vi "RT_Thrust_Force_in_DLR_Body_Reference_System_2 (SubVI).vi"(6 "Act_b(i)":dbl[](array[numeric]), 8 "Vehicle Parameters":T1, 9 "i":i32, 10 "cluster":T2, 11 "Data":dbl[][](array[numeric])) -> (3 "FE_b":dbl[](array[numeric]))   [LabVIEW 2017]
panel:
  out "Fez":dbl
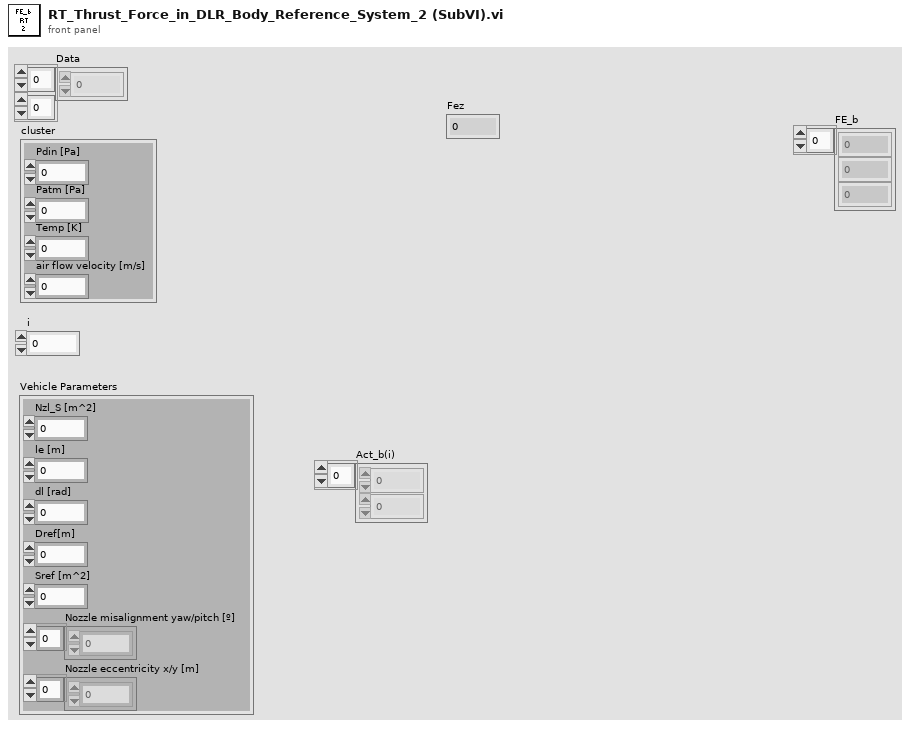
[diagram p1: front panel]
types:
  T1 = cluster{"Nzl_S [m^2]":dbl, "le [m]":dbl, "dl [rad]":dbl, "Dref[m]":dbl, "Sref [m^2]":dbl, "Nozzle misalignment yaw/pitch [º]":dbl[], "Nozzle eccentricity x/y [m]":dbl[]}
  T2 = cluster{"Pdin [Pa]":dbl, "Patm [Pa]":dbl, "Temp [K]":dbl, "air flow velocity [m/s]":dbl}
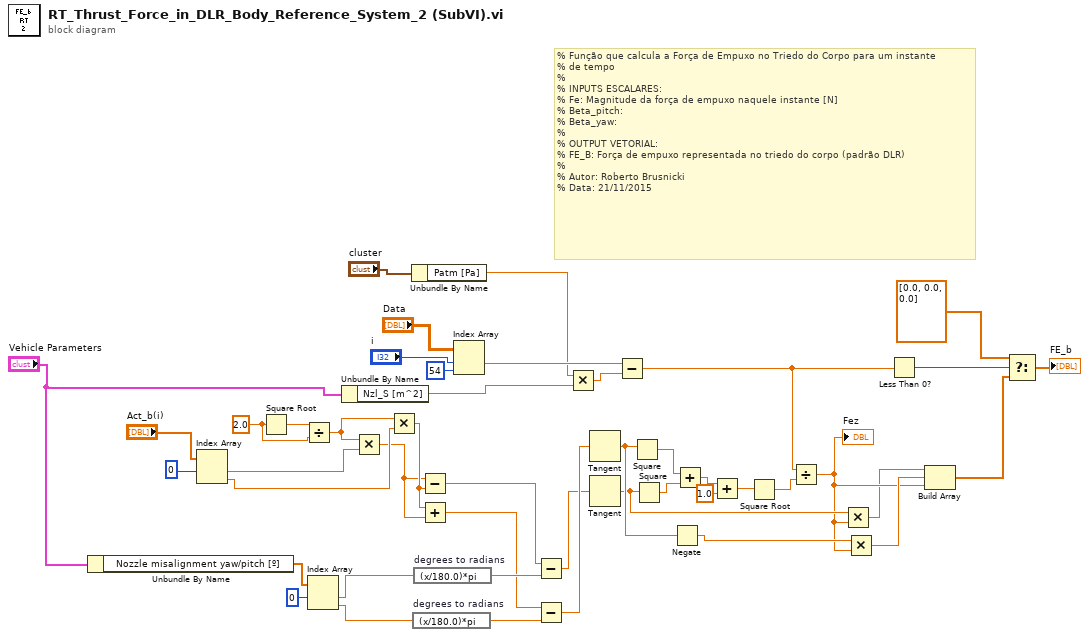
[diagram p0: block diagram]
diagram:
  w19 = 2.0 ("x")
  # "% Função que calcula a Força de Empuxo no Triedo do Corpo para um instante\n% de tempo\n%\n% INPUTS ESCALARES:\n% Fe: Magnitude da força de empuxo naquele instante [N]\n% Beta_pitch: \n% Beta_yaw:\n%\n% OUTPUT VETORIAL:\n% FE_B: Força de empuxo representada no triedo do corpo (padrão DLR)\n%\n% Autor: Roberto Brusnicki\n% Data: 21/11/2015"
  n1 = Unbundle By Name("Vehicle Parameters") -> ("Nozzle misalignment yaw/pitch [º]"=w1:dbl[])
  n2 = Index Array(array="Act_b(i)", index #1=0 ("disabled index (col)")) -> (element #1=w18:dbl, element #2=w16:dbl)  [unwired: 1 in]
  n3 = Square Root(x=w19) -> (sqrt(x)=w20:dbl)
  n4 = Divide(x=w20, y=w19) -> (x/y=w17:dbl)
  n5 = Index Array(array=w1, index #1=0 ("index")) -> (element #1=w4:dbl, element #2=w3:dbl)  [unwired: 1 in]
  n6 = Unbundle By Name("Vehicle Parameters") -> ("Nzl_S [m^2]"=w6:dbl)
  n7 = Multiply(x=w17, y=w18) -> (x*y=w13:dbl)
  n8 = Multiply(x=w17, y=w16) -> (x*y=w14:dbl)
  n9 = Unbundle By Name("cluster") -> ("Patm [Pa]"=w7:dbl)
  n10 = expression code="(x/180.0)*pi" "degrees to radians"(w3) -> (w21:dbl)
  n11 = expression code="(x/180.0)*pi" "degrees to radians"(w4) -> (w22:dbl)
  n12 = Subtract(x=w13, y=w14) -> (x-y=w15:dbl)
  n13 = Add(x=w14, y=w13) -> (x+y=w12:dbl)
  n14 = Index Array(array="Data", index (row)="i", index (col)=54 ("disabled index (col)")) -> (element=w9:dbl)
  n15 = Subtract(x=w15, y=w22) -> (x-y=w10:dbl)
  n16 = Subtract(x=w12, y=w21) -> (x-y=w11:dbl)
  n17 = Multiply(x=w7, y=w6) -> (x*y=w29:dbl)
  n18 = Tangent(1:w11) -> (0:w40:dbl)
  n19 = Tangent(1:w10) -> (0:w39:dbl)
  n20 = Subtract(x=w9, y=w29) -> (x-y=w25:dbl)
  n21 = Square(x=w40) -> (x^2=w32:dbl)
  n22 = Square(x=w39) -> (x^2=w31:dbl)
  n23 = Negate(x=w40) -> (-x=w41:dbl)
  n24 = Add(x=w32, y=w31) -> (x+y=w33:dbl)
  n25 = Add(x=w33, y=1.0) -> (x+y=w35:dbl)
  n26 = Square Root(x=w35) -> (sqrt(x)=w36:dbl)
  n27 = Divide(x=w25, y=w36) -> (x/y=w38:dbl)
  "Fez" <- w38
  n28 = Multiply(x=w39, y=w38) -> (x*y=w37:dbl)
  n29 = Multiply(x=w41, y=w38) -> (x*y=w42:dbl)
  n30 = Less Than 0?(x=w25) -> (x < 0?=w30:bool)
  n31 = Build Array(w37, w42, w38) -> (w44:dbl[])
  n32 = Select(t=dbl[] [0.0, 0.0, 0.0], s=w30, f=w44) -> (s? t:f=→"FE_b":dbl[])
